vi "Test-Wrist.vi"() -> ()   [LabVIEW 2023]
doc: "This VI implements the framework and scheduler for your robotics program. It should not be necessary to modify the framework. You are expected to add your code to the VIs called from Robot Main - the ones located in the Team Code folder within the project."
uses:
  <vilib>/Rock Robotics/WPI/DriverStation/WPI_DriverStationRobotMode2.ctl
  Robot Global Data.vi
  Wrist/WristGlobal.vi
  <vilib>/Rock Robotics/WPI/ThirdParty/JAS_Junk/TrajLib/Trajectory_Library.lvlib
panel:
  in  "Inc":bool
  in  "Dec":bool
  in  "Flat":bool
  in  "Slant":bool
  in  "Cancel":bool
  in  "Rest":bool
  out "Wrist Chart":T1(graph)
  out "Battery_Volts":dbl format="%9.1f"
  out "WristSP Deg":dbl format="%9.1f"
  out "At Low Limit":bool
  out "At High Limit":bool
  out "WristAngle Deg":dbl format="%9.1f"
  out "Robot Mode":T2
  out "MotorOutDmd":dbl format="%9.2f"
  in  "error in (no error)":errorcluster
  in  "Finish":bool
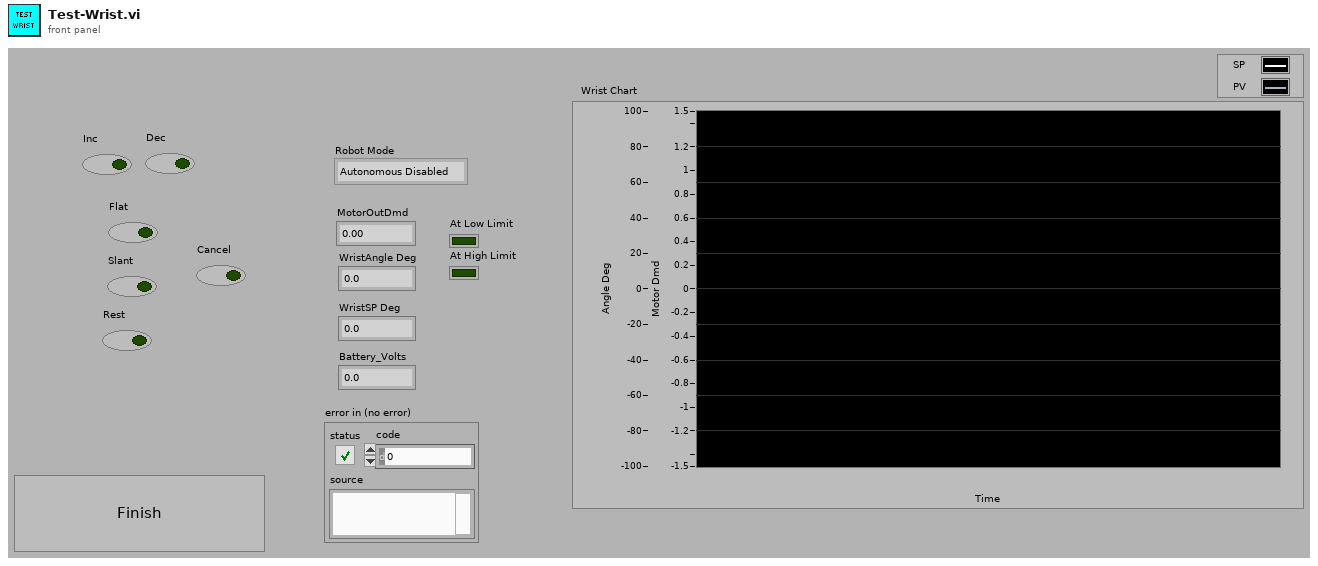
[diagram p1: front panel]
types:
  T1 = cluster{"ElevatorPosDemandHeight":dbl, "ElevHeightInch":dbl, "MotorDemand":dbl}
  T2 = typedef "WPI_DriverStationRobotMode2.ctl" = enum16{"Autonomous Disabled", "Autonomous Enabled", "Teleop Disabled", "Teleop Enabled", "Disconnected", "Finish", "Test Disabled", "Test Enabled", "Emergency Stopped"}
  T3 = cluster{"CurrentWristSetpoint":dbl, "WritstPositionDegrees":dbl, "MotorDmd":dbl}
  T4 = typedef "WPI_DriverStationMatch Info.ctl" = cluster{"Autonomous Elapsed Seconds":dbl, "TeleOp Elapsed Seconds":dbl, "Disabled Elapsed Seconds":dbl, "Visited Autonomous":bool, "Visited TeleOp":bool, "Visited Disabled":bool, "Autonomous Settings":cluster{"Autonomous Style":enum16{"Iterative", "Independent"}, "VI Refnum":refnum<vi>}}
  T5 = typedef "WPI_DriverStationDerivedRobotMode.ctl" = enum16{"Init", "Execute", "Stop"}
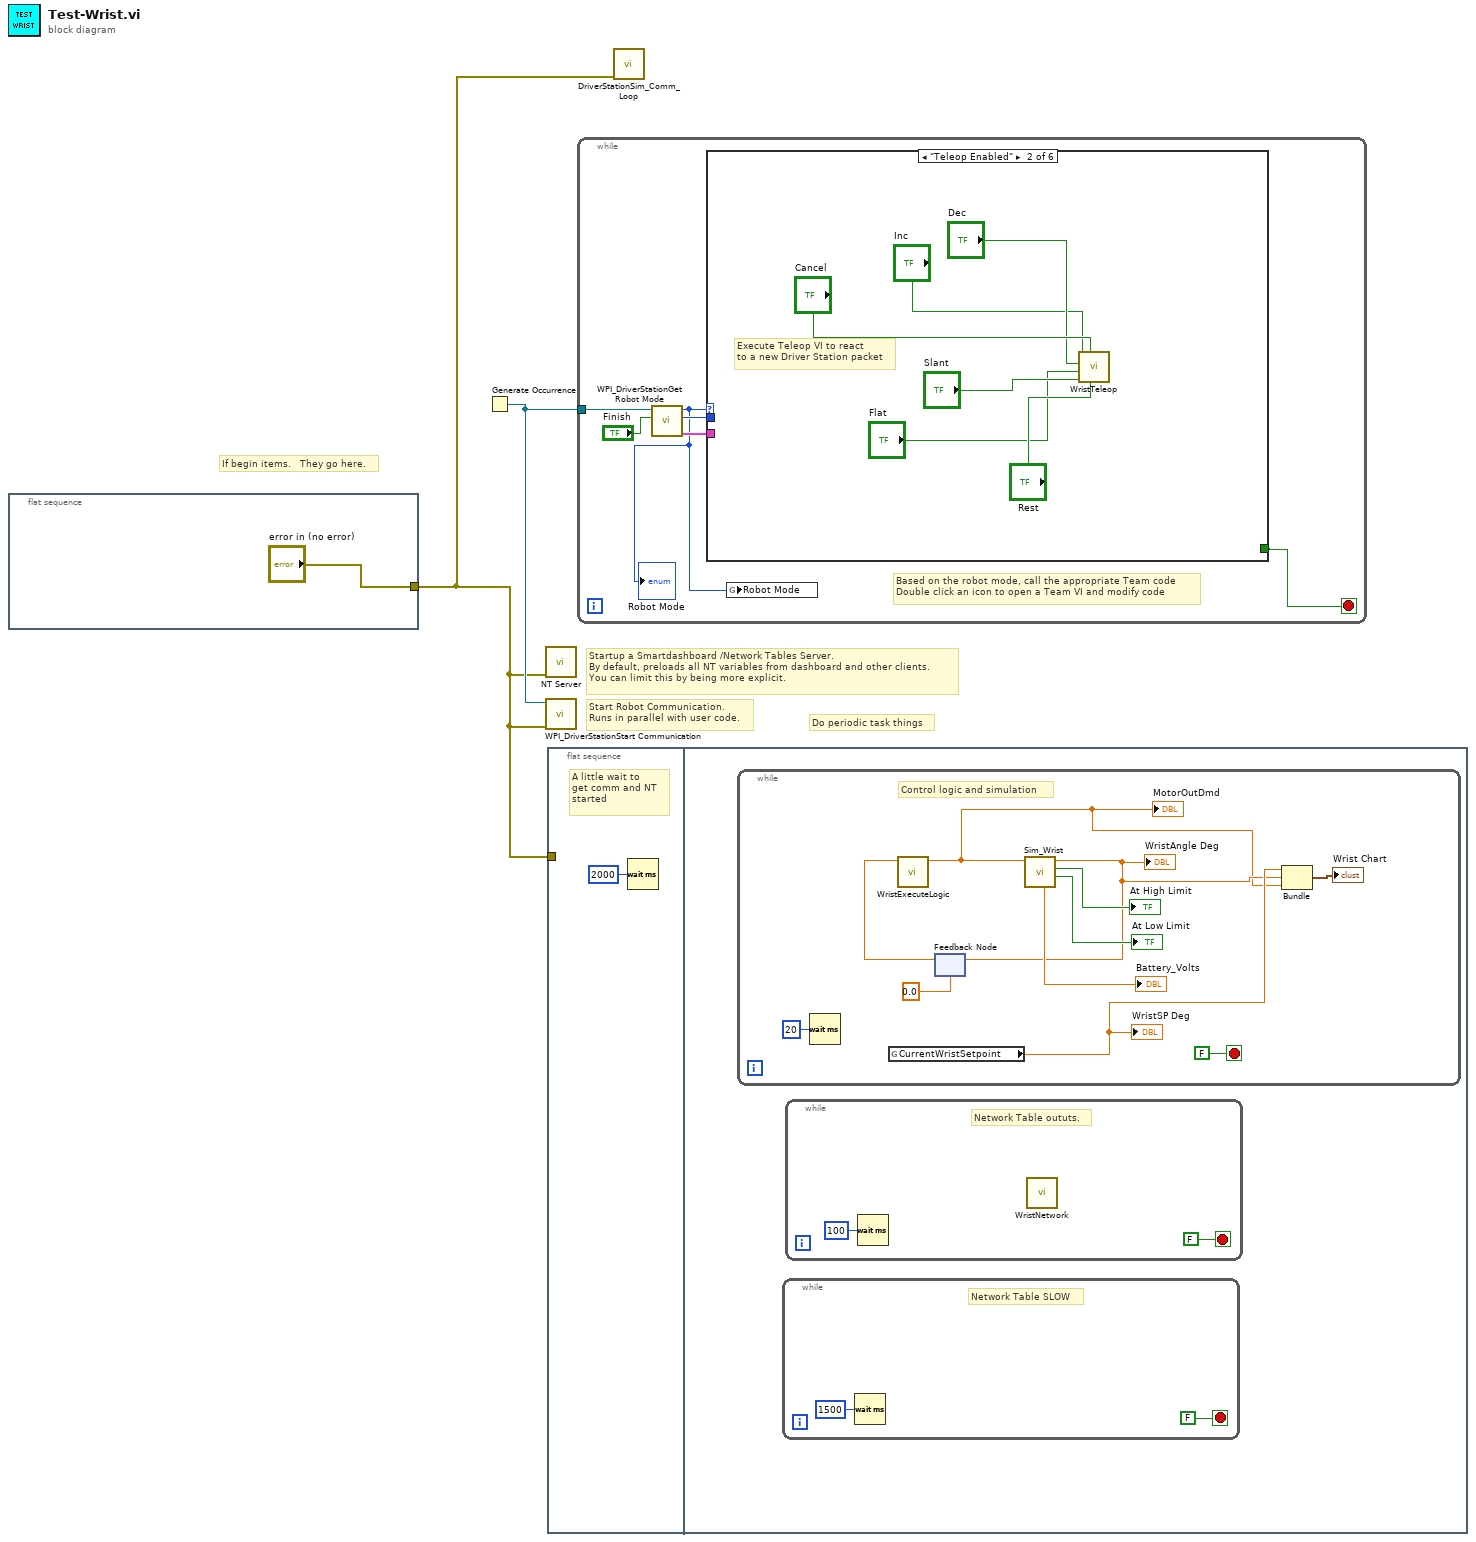
[diagram p0: block diagram]
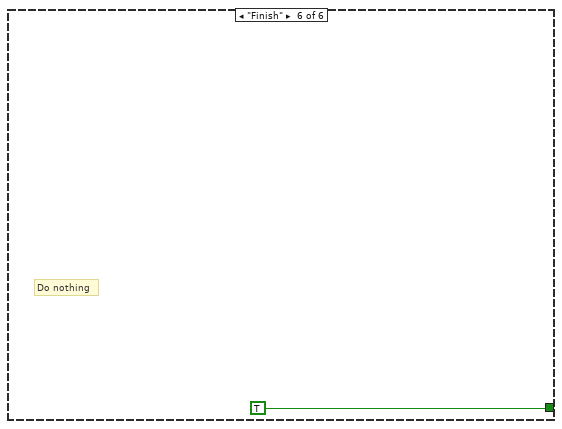
[diagram p6: hidden frame]
diagram:
  # "If begin items.   They go here."
  # "Do periodic task things"
  # "Startup a Smartdashboard /Network Tables Server.\nBy default, preloads all NT variables from dashboard and other clients.\nYou can limit this by being more explicit."
  # "Start Robot Communication.\nRuns in parallel with user code."
  n1 = flat-sequence {
    tunnel: ["error in (no error)"] -> w1
    frame #0 {
    }
  }
  n2 = Generate Occurrence() -> (w2:refnum<k4>)
  n3 = call <vilib>:"NT Server.vi"("error in (no error)"=w1) -> ()  [unwired: 10 in, 1 out]
  n4 = call <vilib>:"WPI_DriverStationStart Communication.vi"("error in (no error)"=w1, "occurrence"=w2) -> ()  [unwired: 1 in, 9 out]
  n5 = flat-sequence {
    tunnel: w1 -> [_]
    frame #0 {
      # "A little wait to\nget comm and NT\nstarted"
      n6 = Wait (ms)(milliseconds to wait=u32 2000) -> ()  [unwired: 1 out]
    }
    frame #1 {
      n7 = while {
        stop <- FALSE stop-if-true
        # "Control logic and simulation"
        n8 = Wait (ms)(milliseconds to wait=u32 20) -> ()  [unwired: 1 out]
        n9 = global read "WristGlobal.vi" "CurrentWristSetpoint"() -> (w12:dbl)
        "WristSP Deg" <- w12
        n10 = feedback #1(0.0 ("WritstPositionDegrees")) -> (w13:dbl)
        n11 = call "WristExecuteLogic.vi"("EncoderPos (deg)"=w13) -> ("MotorDmd"=w9:dbl)  [unwired: 9 in, 1 out]
        "MotorOutDmd" <- w9
        n12 = call "Sim_Wrist.vi"("Motor1 Dmd"=w9) -> ("AtLowLimit"=→"At Low Limit":bool, "At HIgh LImit"=→"At High Limit":bool, "WritstPositionDegrees"=w11:dbl, "Voltage"=→"Battery_Volts":dbl)  [unwired: 6 in, 1 out]
        "WristAngle Deg" <- w11
        n13 = feedback-in #1(w11) -> ()
        n14 = Bundle("CurrentWristSetpoint"=w12, "WritstPositionDegrees"=w11, "MotorDmd"=w9) -> (→"Wrist Chart":T3)  [unwired: 1 in]
      }
      n15 = while {
        stop <- FALSE stop-if-true
        # "Network Table SLOW"
        n16 = Wait (ms)(milliseconds to wait=u32 1500) -> ()  [unwired: 1 out]
      }
      n17 = while {
        stop <- FALSE stop-if-true
        # "Network Table oututs."
        n18 = Wait (ms)(milliseconds to wait=u32 100) -> ()  [unwired: 1 out]
        n19 = call "WristNetwork.vi"() -> ()  [unwired: 12 in]
      }
    }
  }
  n20 = while {
    tunnel: w2 -> [w25]
    stop <- w20 stop-if-true
    # "Based on the robot mode, call the appropriate Team code\nDouble click an icon to open a Team VI and modify code"
    n21 = call <vilib>:"WPI_DriverStationGet Robot Mode.vi"("Finish"="Finish", "DS Occurrence"=w25) -> ("Match Info out"=w22:T4, "Call Context"=w24:T5, "Robot Mode"=w21:T2)  [unwired: 7 out]
    "Robot Mode" <- w21
    n22 = case shown="\"Teleop Enabled\"" w21 {
      tunnel: w24 -> [_ _ _ _ _ _]
      tunnel: w22 -> [_ _ _ _ _ _]
      tunnel: [_ _ _ _ _ TRUE] -> w20
      frame "Autonomous Enabled" {
        # "Do nothing...."
      }
      frame "Teleop Enabled" {
        # "Execute Teleop VI to react\nto a new Driver Station packet"
        n23 = call "WristTeleop.vi"("Rest"="Rest", "Cancel"="Cancel", "Slant"="Slant", "Flat"="Flat", "Dec"="Dec", "Inc"="Inc") -> ()  [unwired: 6 in]
      }
      frame "Test Disabled", "Test Enabled" {
        # "Do nothing"
      }
      frame "Autonomous Disabled", "Teleop Disabled" {
        # "Do nothing."
      }
      frame "Disconnected", Default {
        # "Driver Station packet didn't arrive.\nPossibly useful for diagnostics"
      }
      frame "Finish" {
        # "Do nothing"
      }
    }
    n24 = global write "Robot Global Data.vi" "Robot Mode"(w21) -> ()
  }
  n25 = call <vilib>:"DriverStationSim_Comm_Loop.vi"("error in (no error)"=w1) -> ()  [unwired: 11 in]
